vi "grabberpidinit.vi"(9 "setpoint":dbl format="%.2f", 11 "reinitialize? (F) 2":bool) -> (0 "Done? 2":bool, 2 "output":dbl format="%.2f")   [LabVIEW 2013]
uses:
  <vilib>/addons/control/pid/pid.llb/PID (DBL).vi
  <vilib>/addons/control/pid/NI_PID_pid.lvlib
panel:
  in  "adjuster":dbl
  in  "PID Gains for Angle":T1={"proportional gain (Kc)"=1.2, "integral time (Ti, min)"=0.011, "derivative time (Td, min)"=0.007} {"derivative time (Td, min)" format="%.3f"; "integral time (Ti, min)" format="%.3f"; "proportional gain (Kc)" format="%.3f"}
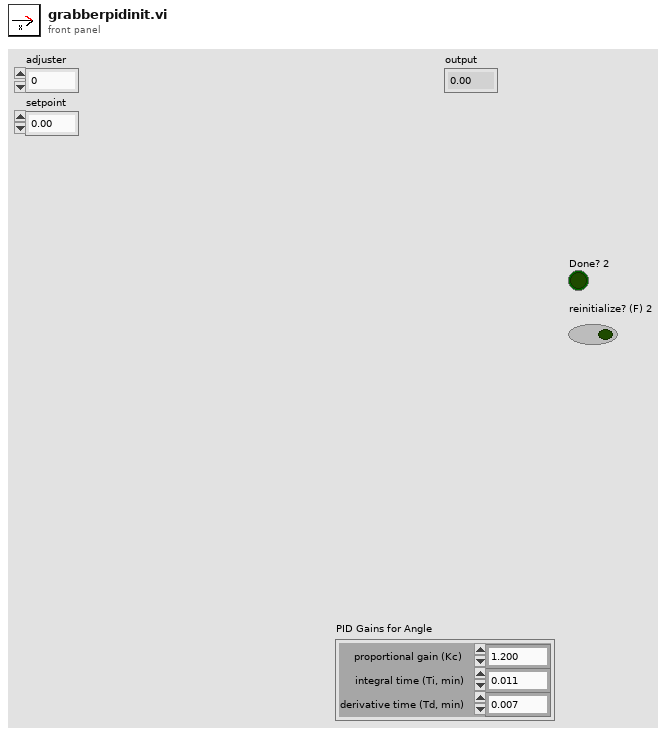
[diagram p1: front panel]
types:
  T1 = cluster{"proportional gain (Kc)":dbl, "integral time (Ti, min)":dbl, "derivative time (Td, min)":dbl}
  T2 = typedef "WPI_EncoderDevRef.ctl" = cluster{"DevStatus":errorcluster, "EncoderIndex":T3, "CounterIndex":T4, "DistancePerCount":dbl, "Decoding Type":T5}
  T3 = typedef "FPGA_EncoderIdx.ctl" = enum8{"Enc 0", "Enc 1", "Enc 2", "Enc 3", "Invalid"}
  T4 = typedef "FPGA_CounterCtrSystemIndex.ctl" = enum8{"Ctr 0", "Ctr 1", "Ctr 2", "Ctr 3", "Ctr 4", "Ctr 5", "Ctr 6", "Ctr 7", "Invalid"}
  T5 = typedef "WPI_EncoderType.ctl" = enum16{"1x", "2x", "4x"}
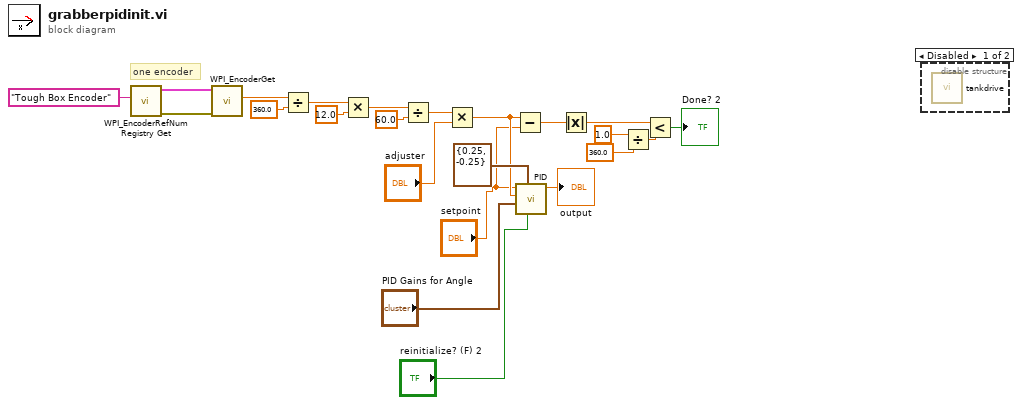
[diagram p0: block diagram]
diagram:
  # "one encoder"
  n1 = call <vilib>:"WPI_EncoderRefNum Registry Get.vi"("refnum name"="Tough Box Encoder") -> ("error out"=w23:errorcluster, "EncoderDevRef"=w22:T2)  [unwired: 9 in]
  n2 = call <vilib>:"WPI_EncoderGet.vi"("error in (no error)"=w23, "EncoderDevRef"=w22) -> ("Distance"=w13:dbl)  [unwired: 4 in, 5 out]
  n3 = Divide(x=w13, y=360.0) -> (x/y=w11:dbl)
  n4 = Multiply(x=w11, y=12.0) -> (x*y=w12:dbl)
  n5 = Divide(x=w12, y=60.0) -> (x/y=w8:dbl)
  n6 = Multiply(x=w8, y="adjuster") -> (x*y=w6:dbl)
  n7 = Subtract(x=w6, y="setpoint") -> (x-y=w18:dbl)
  n8 = call-poly <vilib>:"PID.vi"("reinitialize? (F)"="reinitialize? (F) 2", "output range"=cluster{"output high":dbl, "output low":dbl} {"output high"=0.25, "output low"=-0.25}, "PID gains"="PID Gains for Angle", "process variable"=w6, "setpoint"="setpoint") -> ("output"=→"output":dbl)  [unwired: 5 in, 1 out]
  n9 = Absolute Value(x=w18) -> (abs(x)=w19:dbl)
  n10 = Divide(x=1.0, y=360.0) -> (x/y=w1:dbl)
  n11 = Less?(x=w19, y=w1) -> (x < y?=→"Done? 2":bool)
  n12 = disable-structure shown="Disabled" {
    frame Disabled {
      n13 = call "tankdrive.vi"() -> ()  [unwired: 12 in]
    }
    frame Enabled {
    }
  }
